vi "Configure Continuous Acquisition.vi"(8 "error in (no error)":errorcluster, 10 "Continuous Acquisition Mode (T: Enable)":bool=TRUE, 11 "VISA resource name":refnum<visa-resource-name>) -> (0 "error out":errorcluster, 3 "VISA resource name out":refnum<visa-resource-name>)   [LabVIEW 2017, in "Agilent 6000 Series.lvlib"]
doc: "Configures the instrument to run continuously or to stop after a single configured acquistion.\n\nNote:\n(1) This setting does not occur until the <B>Initiate</B> or <B>Read Waveform</B> VI is called.\n(2) Performing an Autosetup, will put the instrument in continuous acquisition mode."
uses:
  <instrlib>/Agilent 6000 Series/Agilent 6000 Series.lvlib
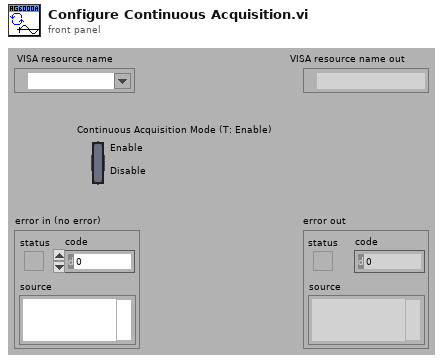
[diagram p1: front panel]
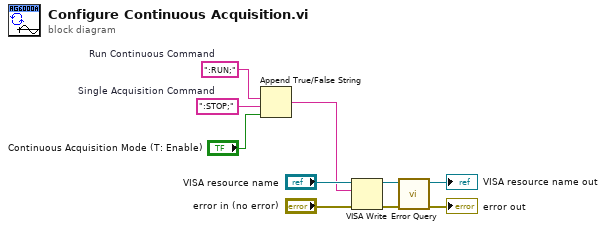
[diagram p0: block diagram]
diagram:
  w3 = ":STOP;"  # Single Acquisition Command
  w4 = ":RUN;"  # Run Continuous Command
  n1 = Append True/False String(1:"Continuous Acquisition Mode (T: Enable)", 2:w3, 3:w4) -> (0:w1:string)  [unwired: 1 in]
  n2 = VISA Write(VISA resource name="VISA resource name", write buffer=w1, error in (no error)="error in (no error)") -> (VISA resource name out=w6:refnum<visa-resource-name>, error out=w5:errorcluster)  [unwired: 1 out]
  n3 = call <instrlib>:"Error Query.vi"("error in (no error)"=w5, "VISA resource name"=w6) -> ("error out"=→"error out":errorcluster, "VISA resource name out"=→"VISA resource name out":refnum<visa-resource-name>)  [unwired: 6 in, 2 out]
